vi "CpStats.vi"(10 "Cp=P/Pdyn":dbl[](array[numeric]), 11 "TapNo":i32) -> (1 "StatsCluster":T1 {"Min" format="%0.2f"; "Max" format="%0.2f"; "mean(5Maxs)" format="%0.2f"; "mean(5Mins)" format="%0.2f"; "SD(Cp)" format="%0.2f"; "meanCp" format="%0.2f"})   [LabVIEW 2011]
uses:
  <vilib>/Analysis/NI_AALBase.lvlib
panel:
  out "5maxs":dbl[](array[numeric])
  out "5mins":dbl[](array[numeric])
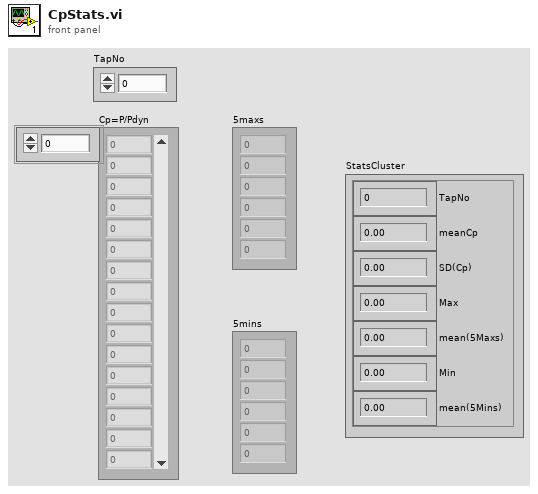
[diagram p1: front panel]
types:
  T1 = cluster{"TapNo":i32, "meanCp":dbl, "SD(Cp)":dbl, "Max":dbl, "mean(5Maxs)":dbl, "Min":dbl, "mean(5Mins)":dbl}
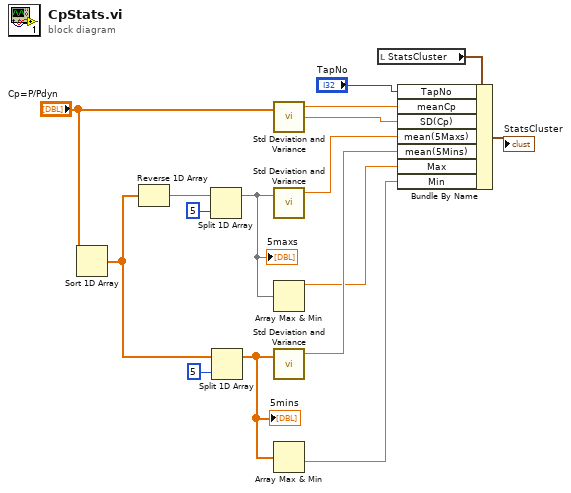
[diagram p0: block diagram]
diagram:
  n1 = Sort 1D Array(array="Cp=P/Pdyn") -> (sorted array=w14:dbl[])
  n2 = Reverse 1D Array(array=w14) -> (reversed array=w12:dbl[])
  n3 = Split 1D Array(array=w12, index=5) -> (first subarray=w9:dbl[])  [unwired: 1 out]
  "5maxs" <- w9
  n4 = Split 1D Array(array=w14, index=5) -> (first subarray=w8:dbl[])  [unwired: 1 out]
  "5mins" <- w8
  n5 = call <vilib>:"Std Deviation and Variance.vi"("X"="Cp=P/Pdyn") -> ("mean"=w7:dbl, "standard deviation"=w6:dbl)  [unwired: 1 in, 1 out]
  n6 = call <vilib>:"Std Deviation and Variance.vi"("X"=w9) -> ("mean"=w5:dbl)  [unwired: 1 in, 2 out]
  n7 = Array Max & Min(array=w9) -> (max value=w3:dbl)  [unwired: 3 out]
  n8 = call <vilib>:"Std Deviation and Variance.vi"("X"=w8) -> ("mean"=w4:dbl)  [unwired: 1 in, 2 out]
  n9 = Array Max & Min(array=w8) -> (min value=w2:dbl)  [unwired: 3 out]
  n10 = local read "StatsCluster"() -> (w10:T1)
  n11 = Bundle By Name(cluster=w10, "TapNo"="TapNo", "meanCp"=w7, "SD(Cp)"=w6, "mean(5Maxs)"=w5, "mean(5Mins)"=w4, "Max"=w3, "Min"=w2) -> (→"StatsCluster":T1)
